vi "RTS Search For Peaks.vi"() -> ()   [LabVIEW 2016]
uses:
  Type Definitions/RTS Macro Full Data.ctl
  Type Definitions/RTS Macro Refrigeration Core Stats.ctl
  <vilib>/ptbypt/NI_PtbyPt.lvlib
  <vilib>/Analysis/NI_AALBase.lvlib
panel:
  out "XY Graph":cluster{"Y":dbl[], "Y":dbl[]}[](graph)
  out "Refrigeration Core Stats":T1 {"Average Compressor Cycle Time (Min)" format="%0.2f"; "Average Compressor Power (W)" format="%0.2f"; "Power Start Time (sec)" format="%<%H:%M:%S>t"; "Power End time (sec)" format="%<%H:%M:%S>t"; "Average Defrost Power (W)" format="%0.2f"}
  in  "Full Refrigeration Data":T2
  in  "Error In":errorcluster
  out "Locations":i32[](array[numeric])
  out "Waveform Graph 7":i32[](graph)
  out "Waveform Graph 6":i32[](graph)
  out "Waveform Graph 4":i32[](graph)
  out "Waveform Graph":waveform(dbl)(graph)
  out "deleted portion":string[][](array[string])
  out "all rows":string[][](array[string])
  in  "Path":path
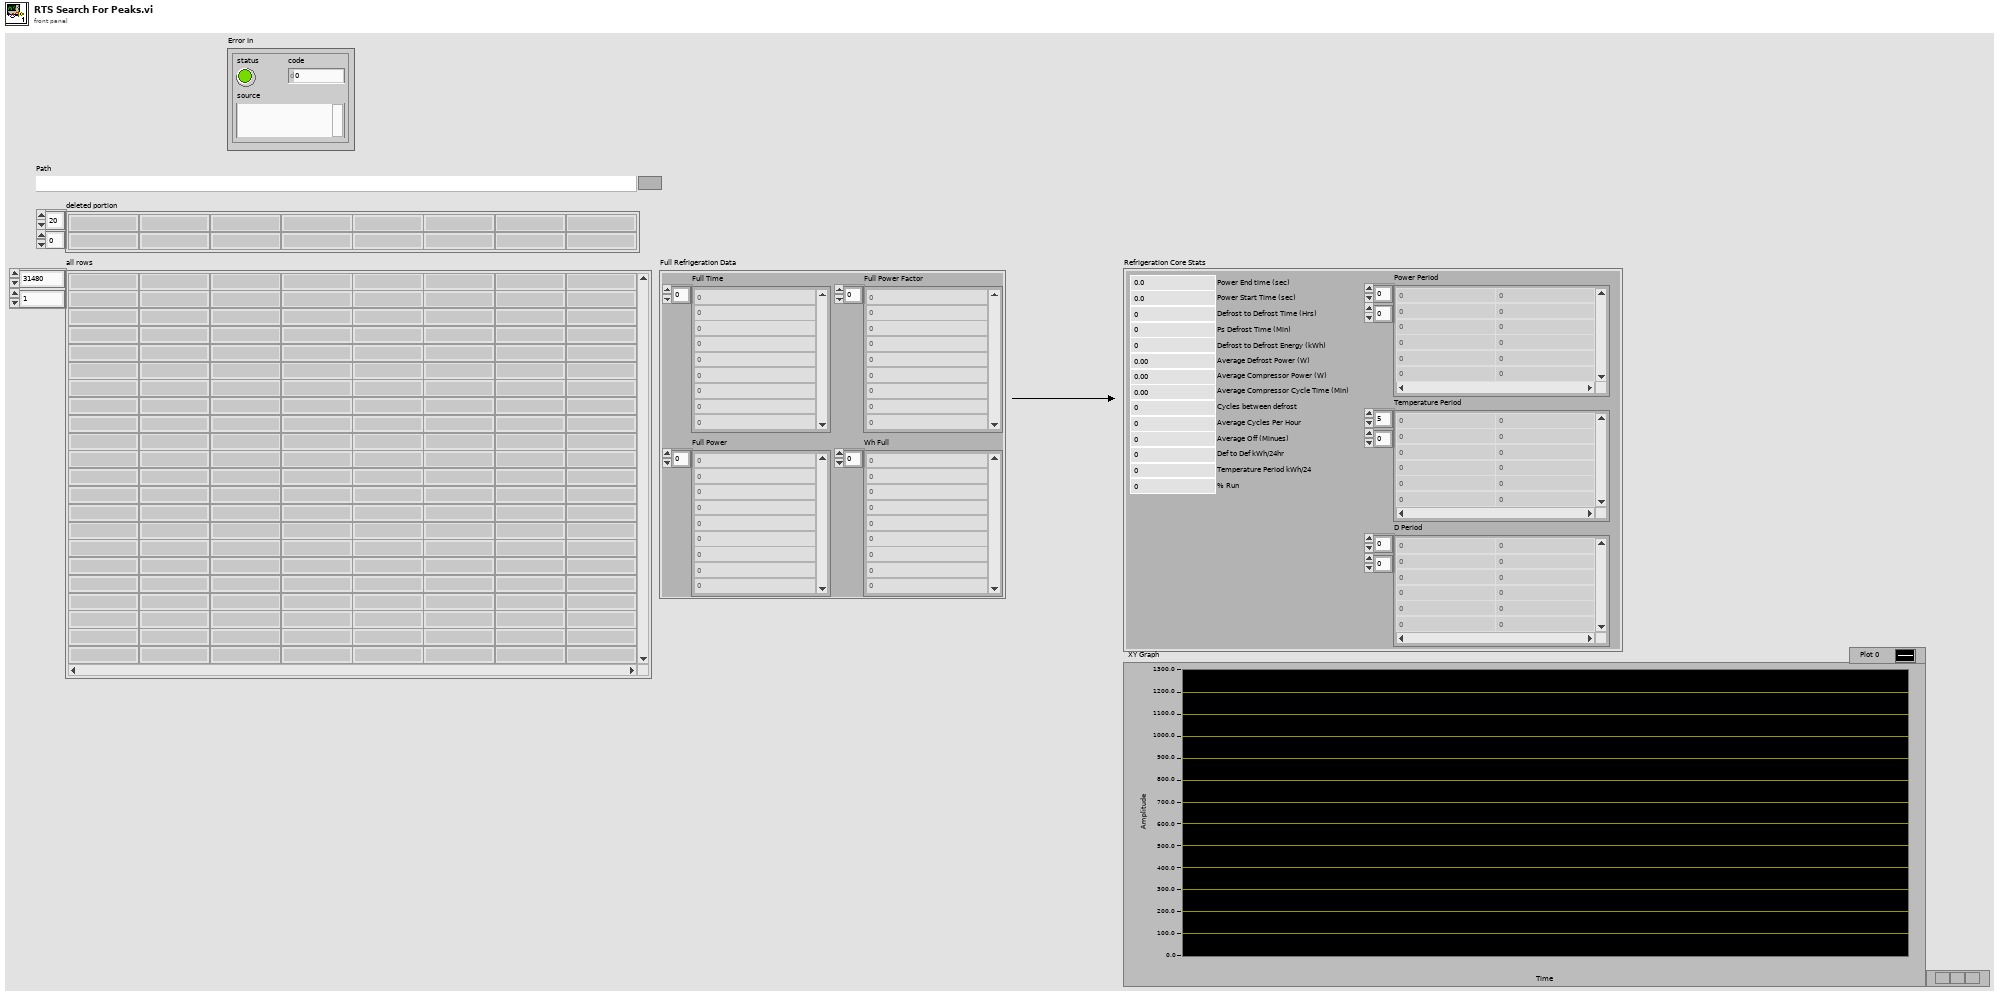
[diagram p1: front panel]
types:
  T1 = typedef "RTS Macro Refrigeration Core Stats.ctl" = cluster{"Average Defrost Power (W)":dbl, "Power End time (sec)":dbl, "Power Start Time (sec)":dbl, "Defrost to Defrost Time (Hrs)":dbl, "Ps Defrost Time (Min)":dbl, "Defrost to Defrost Energy (kWh)":dbl, "Average Compressor Power (W)":dbl, "Average Compressor Cycle Time (Min)":dbl, "Power Period":dbl[][], "Cycles between defrost":i32, "Average Cycles Per Hour":dbl, "Average Off (Minues)":dbl, "Def to Def kWh/24hr":dbl, "Temperature Period kWh/24":dbl, "% Run":dbl, "Temperature Period":dbl[][], "D Period":dbl[][]}
  T2 = typedef "RTS Macro Full Data.ctl" = cluster{"Full Time":dbl[], "Full Power Factor":dbl[], "Full Power":dbl[], "Wh Full":dbl[]}
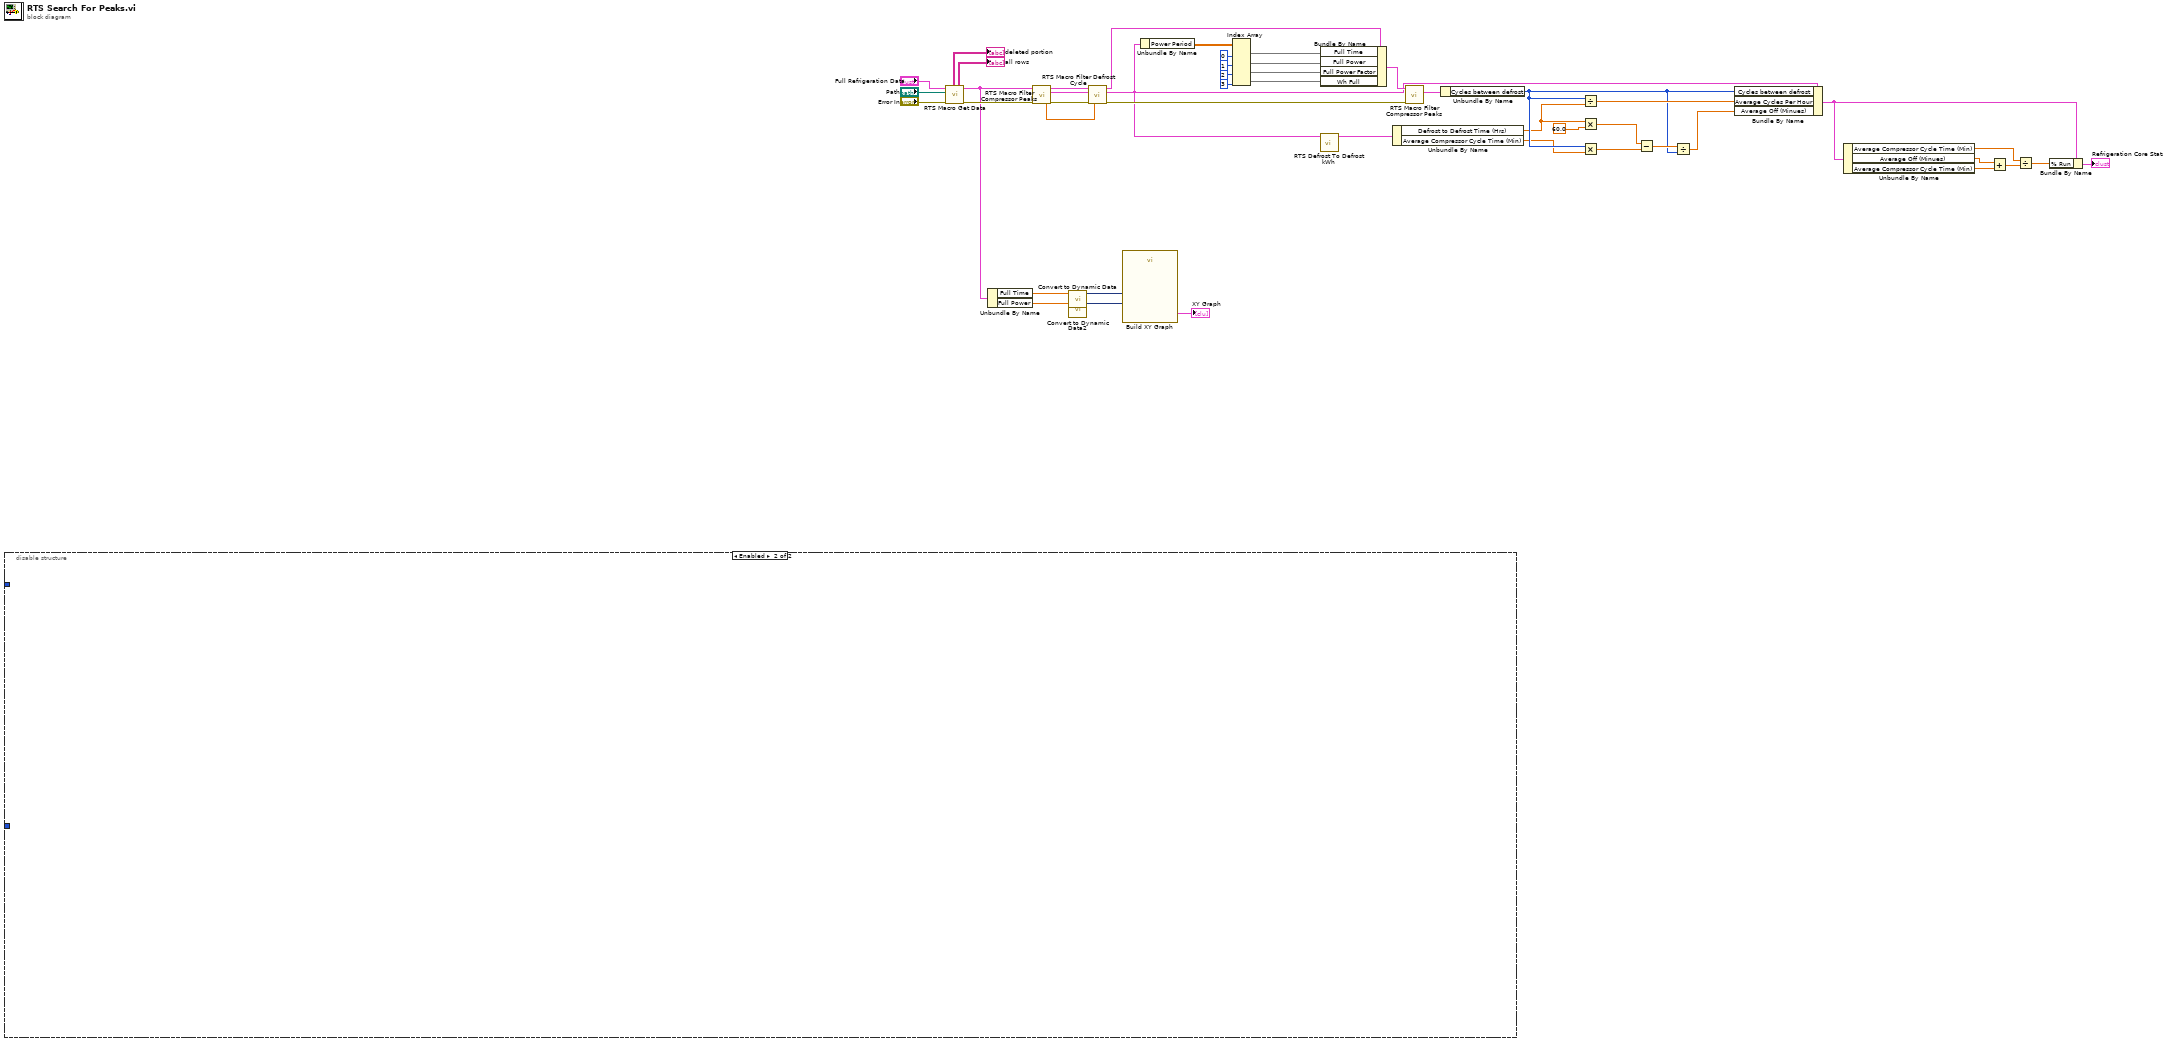
[diagram p0: block diagram]
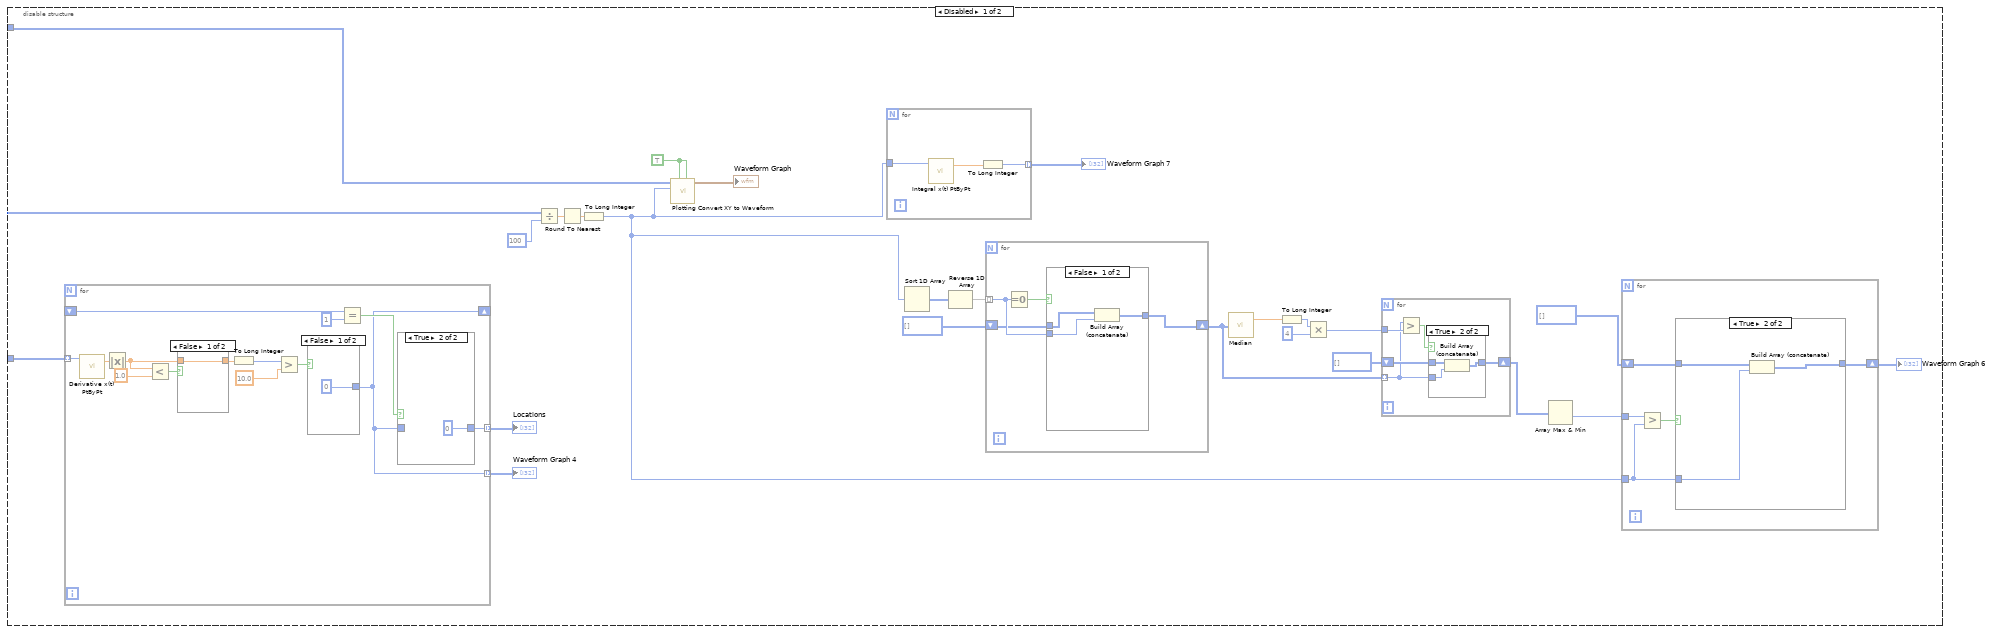
[diagram p2: hidden frame]
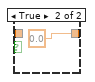
[diagram p7: hidden frame]
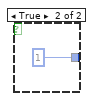
[diagram p8: hidden frame]
diagram:
  n1 = disable-structure shown="Enabled" {
    disable-tunnel: _ -> [w67 _]
    disable-tunnel: _ -> [w52 _]
    frame Disabled {
      w71 = TRUE ("Use Filter?")
      n2 = for {
        tunnel: w67 -> [w114] mode=indexing
        tunnel: [w102] -> w48 mode=indexing
        shift-right: [w101] -> _
        shift-left: _ -> [w105]
        tunnel: [w101] -> w69 mode=indexing
        n3 = call <vilib>:"Derivative x(t) PtByPt.vi"("x"=w114) -> ("dx/dt"=w113:dbl)  [unwired: 3 in, 1 out]
        n4 = Absolute Value(x=w113) -> (abs(x)=w107:dbl)
        n5 = Less?(x=w107, y=1.0) -> (x < y?=w108:bool)
        n6 = case shown="False" w108 {
          tunnel: w107 -> [w117 _]
          tunnel: [w117 0.0 ("y")] -> w106
          frame False {
          }
          frame True {
          }
        }
        n7 = To Long Integer(number=w106) -> (32bit integer=w110:i32)
        n8 = Greater?(x=w110, y=10.0) -> (0:w111:bool)
        n9 = case shown="False" w111 {
          tunnel: [0 1] -> w101
          frame False {
          }
          frame True {
          }
        }
        n10 = Equal?(x=w105, y=1) -> (x = y?=w103:bool)
        n11 = case shown="True" w103 {
          tunnel: w101 -> [w115 _]
          tunnel: [w115 0] -> w102
          frame False {
          }
          frame True {
          }
        }
      }
      "Waveform Graph 4" <- w69
      "Locations" <- w48
      n12 = Divide(x=w67, y=100) -> (x/y=w66:dbl)
      n13 = Round To Nearest(number=w66) -> (nearest integer value=w65:dbl)
      n14 = To Long Integer(number=w65) -> (32bit integer=w49:i32)
      n15 = call "Plotting Convert XY to Waveform.vi"("Macro Filter"=w71, "Use Filter?"=w71, "Y"=w49, "X"=w52) -> ("Waveform Graph"=→"Waveform Graph":waveform(dbl))  [unwired: 5 in, 2 out]
      n16 = for {
        tunnel: w49 -> [w74]
        tunnel: [w72] -> w50 mode=indexing
        n17 = call <vilib>:"Integral x(t) PtByPt.vi"("x"=w74) -> ("integral x(t)"=w73:dbl)  [unwired: 3 in, 1 out]
        n18 = To Long Integer(number=w73) -> (32bit integer=w72:i32)
      }
      "Waveform Graph 7" <- w50
      n19 = Sort 1D Array(array=w49) -> (sorted array=w64:i32[])
      n20 = Reverse 1D Array(array=w64) -> (reversed array=w63:i32[])
      n21 = for {
        tunnel: w63 -> [w96] mode=indexing
        shift-right: [w93] -> w57
        shift-left: i32[] [] -> [w95]
        n22 = Equal To 0?(x=w96) -> (x = 0?=w94:bool)
        n23 = case shown="False" w94 {
          tunnel: w96 -> [w99 _]
          tunnel: w95 -> [w98 w100]
          tunnel: [w97 w100] -> w93
          frame False {
            n24 = Build Array (concatenate)(w98, w99) -> (w97:i32[])
          }
          frame True {
          }
        }
      }
      n25 = call <vilib>:"Median.vi"("X"=w57) -> ("median"=w61:dbl)  [unwired: 1 out]
      n26 = To Long Integer(number=w61) -> (32bit integer=w60:i32)
      n27 = Multiply(x=w60, y=4) -> (x*y=w58:i32)
      n28 = for {
        tunnel: w58 -> [w88]
        tunnel: w57 -> [w84] mode=indexing
        shift-right: [w85] -> w54
        shift-left: i32[] [] -> [w86]
        n29 = Greater?(x=w84, y=w88) -> (0:w87:bool)
        n30 = case shown="True" w87 {
          tunnel: w86 -> [w89 w92]
          tunnel: [w89 w91] -> w85
          tunnel: w84 -> [_ w90]
          frame False {
          }
          frame True {
            n31 = Build Array (concatenate)(w92, w90) -> (w91:i32[])
          }
        }
      }
      n32 = Array Max & Min(array=w54) -> (min value=w53:i32)  [unwired: 3 out]
      n33 = for {
        tunnel: w49 -> [w76]
        tunnel: w53 -> [w78]
        shift-right: [w75] -> w51
        shift-left: i32[] [] -> [w79]
        n34 = Greater?(x=w78, y=w76) -> (0:w77:bool)
        n35 = case shown="True" w77 {
          tunnel: w79 -> [w80 w83]
          tunnel: w76 -> [_ w82]
          tunnel: [w80 w81] -> w75
          frame False {
          }
          frame True {
            n36 = Build Array (concatenate)(w83, w82) -> (w81:i32[])
          }
        }
      }
      "Waveform Graph 6" <- w51
    }
    frame Enabled {
    }
  }
  n37 = call "RTS Macro Get Data.vi"("Error In"="Error In", "Path"="Path", "Full Refrigeration Data"="Full Refrigeration Data") -> ("Error Out"=w40:errorcluster, "Refrigeration Full Data Output"=w37:T2, "all rows"=→"all rows":string[][], "deleted portion"=→"deleted portion":string[][])  [unwired: 5 in]
  n38 = Unbundle By Name(w37) -> ("Full Time"=w9:dbl[], "Full Power"=w7:dbl[])
  n39 = call "RTS Macro Filter Compressor Peaks.vi"("Refrigeration Full Data"=w37, "Error In"=w40) -> ("Refrigeration Full Data Output"=w39:T2, "Refrigeration Core Stats"=w38:T1, "Average Compressor Power (Lower)"=w45:dbl, "Error Out"=w46:errorcluster)  [unwired: 9 in, 1 out]
  n40 = call "Convert to Dynamic Data"("Array"=w9) -> ("Dynamic Data Type"=w8:dynamicdata)  [unwired: 3 in]
  n41 = call "Convert to Dynamic Data2"("Array"=w7) -> ("Dynamic Data Type"=w6:dynamicdata)  [unwired: 3 in]
  n42 = call "RTS Macro Filter Defrost Cycle.vi"("Refrigeration Full Data"=w39, "Refrigeration Core Stats Input"=w38, "Error In"=w46, "Average Compressor Power (Lower)"=w45) -> ("Refrigeration Full Data Output"=w25:T2, "Refrigeration Core Stats"=w4:T1, "Error Out"=w35:errorcluster)  [unwired: 9 in]
  n43 = call "Build XY Graph"("Y Input"=w6, "X Input"=w8) -> ("XY Graph"=→"XY Graph":cluster{"X":dbl[], "Y":dbl[]}[])  [unwired: 8 in, 1 out]
  n44 = Unbundle By Name(w4) -> ("Power Period"=w34:dbl[][])
  n45 = Index Array(array=w34, index (col) #1=0 ("disabled index (col)"), index (col) #2=1 ("index (col)"), index (col) #3=2 ("index (col)"), index (col) #4=3 ("index (col)")) -> (element #1=w29:dbl[], element #2=w28:dbl[], element #3=w27:dbl[], element #4=w26:dbl[])  [unwired: 4 in]
  n46 = call "RTS Defrost To Defrost kWh.vi"("Refrigeration Core Stats"=w4) -> ("Refrigeration Core Stats Out"=w1:T1)  [unwired: 9 in, 1 out]
  n47 = Bundle By Name(cluster=w25, "Full Time"=w29, "Full Power"=w28, "Full Power Factor"=w27, "Wh Full"=w26) -> (w36:T2)
  n48 = Unbundle By Name(w1) -> ("Defrost to Defrost Time (Hrs)"=w3:dbl, "Average Compressor Cycle Time (Min)"=w2:dbl)
  n49 = call "RTS Macro Filter Compressor Peaks.vi"("Refrigeration Full Data"=w36, "Error In"=w35) -> ("Refrigeration Core Stats"=w24:T1)  [unwired: 9 in, 4 out]
  n50 = Unbundle By Name(w24) -> ("Cycles between defrost"=w19:i32)
  n51 = Divide(x=w19, y=w3) -> (x/y=w23:dbl)
  n52 = Multiply(x=w3, y=60.0) -> (x*y=w5:dbl)
  n53 = Multiply(x=w19, y=w2) -> (x*y=w21:dbl)
  n54 = Subtract(x=w5, y=w21) -> (x-y=w20:dbl)
  n55 = Divide(x=w20, y=w19) -> (x/y=w18:dbl)
  n56 = Bundle By Name(cluster=w4, "Cycles between defrost"=w19, "Average Cycles Per Hour"=w23, "Average Off (Minues)"=w18) -> (w17:T1)
  n57 = Unbundle By Name(w17) -> ("Average Compressor Cycle Time (Min)"=w12:dbl, "Average Off (Minues)"=w15:dbl, "Average Compressor Cycle Time (Min)"=w14:dbl)
  n58 = Add(x=w15, y=w14) -> (x+y=w13:dbl)
  n59 = Divide(x=w12, y=w13) -> (x/y=w11:dbl)
  n60 = Bundle By Name(cluster=w17, "% Run"=w11) -> (→"Refrigeration Core Stats":T1)
